vi "XY Graph.vi"() -> ()   [LabVIEW 2020]
panel:
  out "(X and Y arrays) Multi Plot":cluster{i32[], dbl[]}[](graph)
  out "(X and Y arrays) Single Plot":cluster{i32[], dbl[]}(graph)
  out "(Array of Pts) Single Plot":cluster{i32, dbl}[](graph)
  out "(Array of Pts) Multi Plot":cluster{cluster{i32, dbl}[]}[](graph)
  # "ÿa\tÿ"
  # "ÿb\tÿ"
  # "ÿc\tÿ"
  # "ÿd\tÿ"
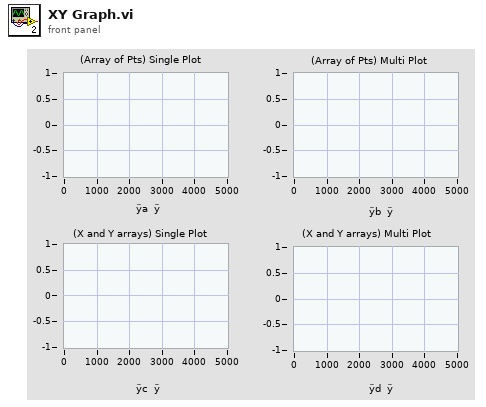
[diagram p1: front panel]
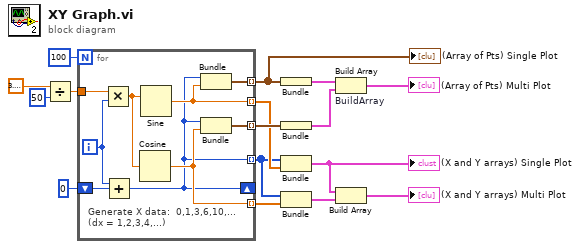
[diagram p0: block diagram]
diagram:
  n1 = Divide(x=3.141592653589793, y=50) -> (x/y=w14:dbl)
  n2 = for {
    N: 100 ("# of Pts") -> [_]
    tunnel: w14 -> [w24]
    shift-right: [w17] -> _
    shift-left: 0 -> [w25]
    tunnel: [w20] -> w9 mode=indexing
    tunnel: [w21] -> w8 mode=indexing
    tunnel: [w19] -> w4 mode=indexing
    tunnel: [w18] -> w12 mode=indexing
    tunnel: [w17] -> w7 mode=indexing
    i -> [w23]
    # "Generate X data:  0,1,3,6,10,...\n(dx = 1,2,3,4,...)"
    n3 = Multiply(x=w24, y=w23) -> (x*y=w22:dbl)
    n4 = Add(x=w23, y=w25) -> (x+y=w17:i32)
    n5 = Cosine(x=w22) -> (cos(x)=w21:dbl)
    n6 = Sine(x=w22) -> (sin(x)=w20:dbl)
    n7 = Bundle "Bundle"(w17, w20) -> (w19:cluster{i32, dbl})  [unwired: 1 in]
    n8 = Bundle "Bundle"(w17, w21) -> (w18:cluster{i32, dbl})  [unwired: 1 in]
  }
  "(Array of Pts) Single Plot" <- w4
  n9 = Bundle "Bundle"(w4) -> (w10:cluster{cluster{i32, dbl}[]})  [unwired: 1 in]
  n10 = Bundle(w12) -> (w11:cluster{cluster{i32, dbl}[]})  [unwired: 1 in]
  n11 = Bundle "Bundle"(w7, w9) -> (w2:cluster{i32[], dbl[]})  [unwired: 1 in]
  "(X and Y arrays) Single Plot" <- w2
  n12 = Bundle "Bundle"(w7, w8) -> (w6:cluster{i32[], dbl[]})  [unwired: 1 in]
  n13 = Build Array "BuildArray"(w10, w11) -> (→"(Array of Pts) Multi Plot":cluster{cluster{i32, dbl}[]}[])
  n14 = Build Array(w2, w6) -> (→"(X and Y arrays) Multi Plot":cluster{i32[], dbl[]}[])
